vi "Test.vi"(0 "Traverse Algorithm in":refnum<class "Build Array.lvclass">, 5 "Terminal To Identify":refnum<vi>, 11 "error in (no error)":errorcluster) -> (4 "Traverse Algorithm out":refnum<class "Build Array.lvclass">, 6 "Terminal for Traversal Continuation":refnum<vi>[](array[refnum]), 8 "Node Identified":bool, 15 "error out":errorcluster)   [LabVIEW 2019, in "MVA Message Mapper.lvlib" / "Build Array.lvclass"]
uses:
  <vilib>/gpm_packages/@cs/Bus-message-mapper/Source/support/Build Array Test/Build Array.lvclass
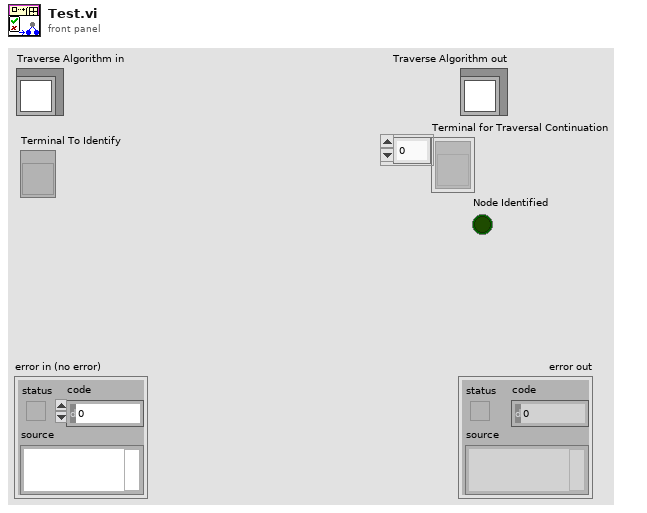
[diagram p1: front panel]
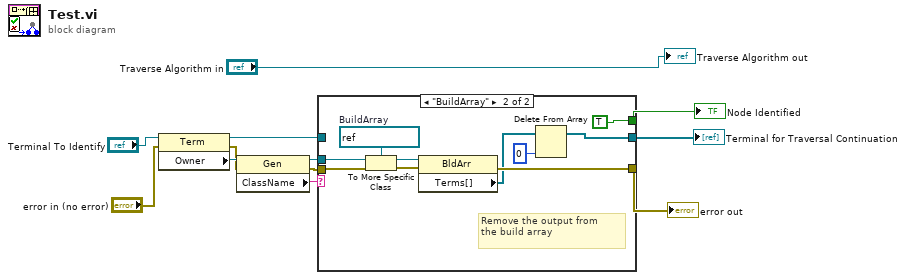
[diagram p0: block diagram]
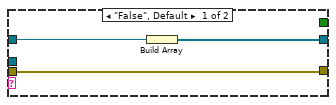
[diagram p2: hidden frame]
diagram:
  n1 = property on="Property Node" class="Term"(reference="Terminal To Identify", error in="error in (no error)") -> (reference out=w10:refnum<vi>, error out=w8:errorcluster, "Owner"=w12:refnum<vi>)
  n2 = property on="Property Node" class="Gen"(reference=w12, error in=w8) -> (reference out=w9:refnum<vi>, error out=w7:errorcluster, "ClassName"=w11:string)
  n3 = case shown="\"BuildArray\"" w11 {
    tunnel: w10 -> [w15 _]
    tunnel: [w13 w17] -> w2
    tunnel: [_ TRUE ("Node Identified")] -> w5
    tunnel: w9 -> [_ w24]
    tunnel: w7 -> [w14 w21]
    tunnel: [w14 w19] -> w1
    frame "False", Default {
      n4 = Build Array(w15) -> (w13:refnum<vi>[])
    }
    frame "BuildArray" {
      w23 = refnum<vi> refnum  # BuildArray
      # "Remove the output from\nthe build array"
      n5 = To More Specific Class(target class=w23, reference=w24, error in=w21) -> (specific class reference=w22:refnum<vi>, error out=w20:errorcluster)
      n6 = property class="BldArr"(reference=w22, error in=w20) -> (error out=w19:errorcluster, "Terms[]"=w18:refnum<vi>[])  [unwired: 1 out]
      n7 = Delete From Array(array=w18, index=0) -> (array with subset deleted=w17:refnum<vi>[])  [unwired: 1 in, 1 out]
    }
  }
  "error out" <- w1
  "Node Identified" <- w5
  "Terminal for Traversal Continuation" <- w2
  "Traverse Algorithm out" <- "Traverse Algorithm in"
